vi "MongoDB.FindAllUsers.vi"(8 "error in (no error)":errorcluster, 11 "MongoDB.Database in":refnum<class "MongoDB.Database.lvclass">) -> (0 "error out":errorcluster, 2 "UserNames":string[](array[string]), 3 "MongoDB.Database out":refnum<class "MongoDB.Database.lvclass">)   [LabVIEW 2014, in "MongoDB.Database.lvclass"]
uses:
  MongoDB.Database.lvclass
  MongoDB.Database.lvclass/MongoDB.Database.ctl
  C:/Users/Richard/Documents/GitHub/mongo-labview-driver/CSharp/bin/MongoDB.Driver.Legacy.dll
  CSharp/bin/MongoDB.Driver.Legacy.dll
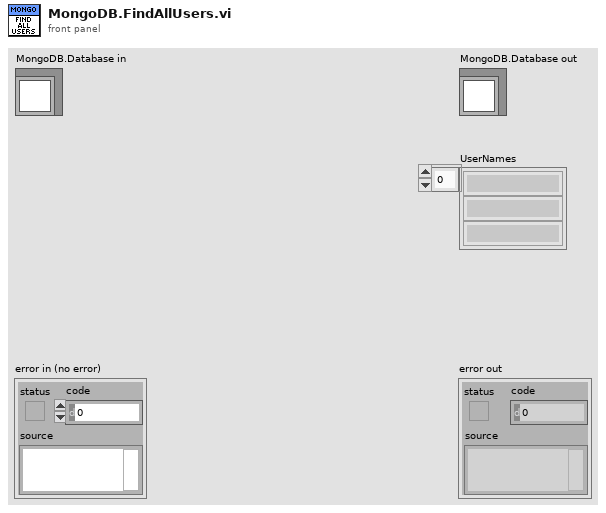
[diagram p1: front panel]
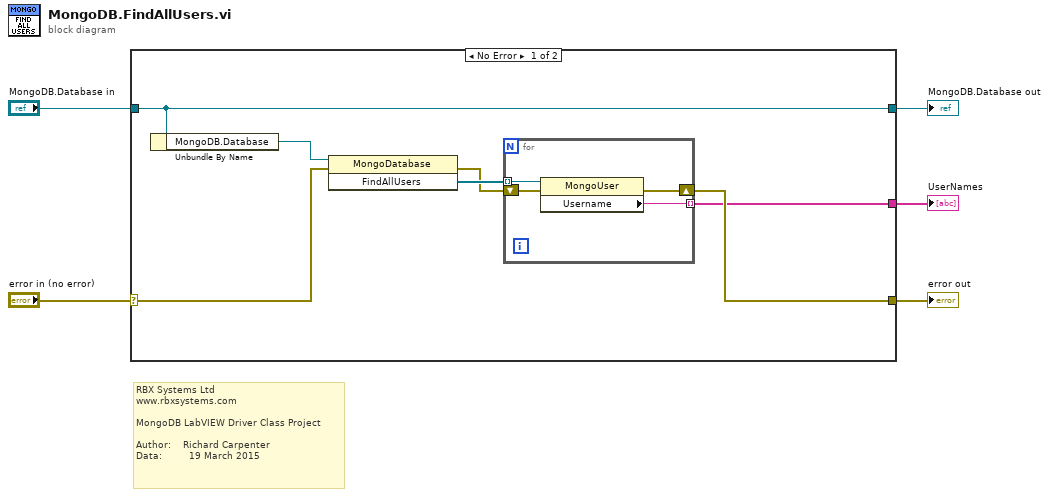
[diagram p0: block diagram]
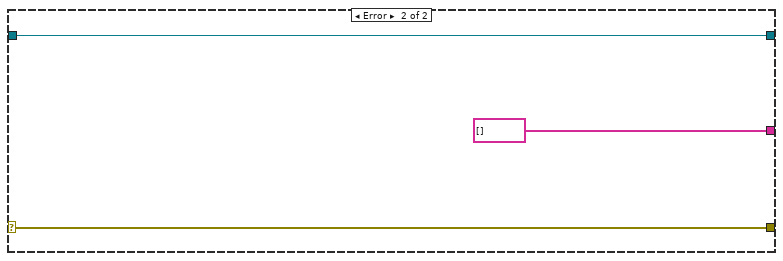
[diagram p2: hidden frame]
diagram:
  # "RBX Systems Ltd\nwww.rbxsystems.com\n\nMongoDB LabVIEW Driver Class Project\n\nAuthor:    Richard Carpenter\nData:         19 March 2015"
  n1 = case shown="No Error" "error in (no error)" {
    selector: "error in (no error)" -> [w6 w19]
    tunnel: [w8 w19] -> w4
    tunnel: [w10 w18] -> w2
    tunnel: "MongoDB.Database in" -> [w10 w18]
    tunnel: [w7 string[] []] -> w1
    frame No Error {
      n2 = Unbundle By Name(w10) -> ("MongoDB.Database"=w9:refnum<k24>)
      n3 = invoke class="MongoDatabase" method="FindAllUsers"(reference=w9, error in=w6) -> (error out=w11:errorcluster, "FindAllUsers"=w12:refnum<k24>[])  [unwired: 1 in, 1 out]
      n4 = for {
        tunnel: w12 -> [w16] mode=indexing
        tunnel: [w15] -> w7 mode=indexing
        shift-right: [w13] -> w8
        shift-left: w11 -> [w14]
        n5 = property class="MongoUser"(reference=w16, error in=w14) -> (error out=w13:errorcluster, "Username"=w15:string)  [unwired: 1 out]
      }
    }
    frame Error {
    }
  }
  "error out" <- w4
  "MongoDB.Database out" <- w2
  "UserNames" <- w1
